vi "RTReedSwitch (1).vi"(8 "error in (no error)":errorcluster) -> (0 "error out":errorcluster)   [LabVIEW 2017]
uses:
  LoopPeriodGLOBAL.vi
  RTControl/StopGLOBAL.vi
  ReedSwitchDistanceGlobal.vi
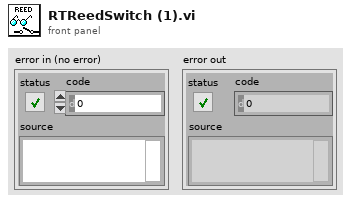
[diagram p1: front panel]
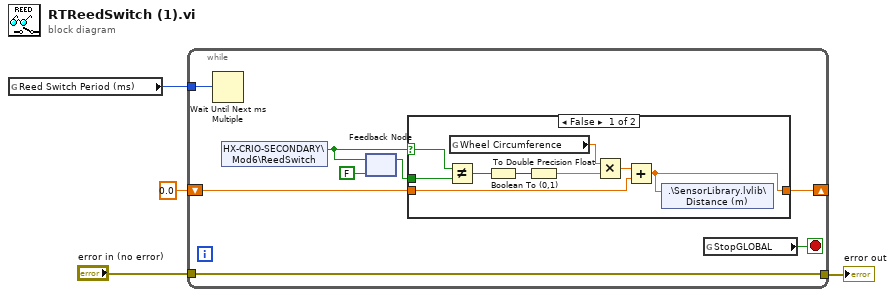
[diagram p0: block diagram]
diagram:
  n1 = global read "LoopPeriodGLOBAL.vi" "Reed Switch Period (ms)"() -> (w1:u32)
  n2 = while {
    shift-right: [w8] -> _
    shift-left: 0.0 -> [w12]
    tunnel: "error in (no error)" -> [w6]
    tunnel: [w6] -> w2
    tunnel: w1 -> [w5]
    stop <- w7 stop-if-true
    n3 = Wait Until Next ms Multiple(millisecond multiple=w5) -> ()  [unwired: 1 out]
    n4 = shared-variable "HX-CRIO-SECONDARY\\Mod6\\ReedSwitch"() -> (w11:bool)  [unwired: 1 in, 1 out]
    n5 = feedback-in #1(w11) -> ()
    n6 = feedback #1(FALSE) -> (w9:bool)
    n7 = case shown="False" w11 {
      selector: w11 -> [w21 _]
      tunnel: w12 -> [w16 w22]
      tunnel: w9 -> [w20 _]
      tunnel: [w13 w22] -> w8
      frame False {
        n8 = Not Equal?(x=w21, y=w20) -> (x != y?=w19:bool)
        n9 = global read "ReedSwitchDistanceGlobal.vi" "Wheel Circumference"() -> (w14:dbl)
        n10 = Boolean To (0,1)(Boolean=w19) -> (0, 1=w18:i16)
        n11 = To Double Precision Float(number=w18) -> (double precision float=w17:dbl)
        n12 = Multiply(x=w14, y=w17) -> (x*y=w15:dbl)
        n13 = Add(x=w15, y=w16) -> (x+y=w13:dbl)
        n14 = shared-variable ".\\SensorLibrary.lvlib\\Distance (m)"(w13) -> ()  [unwired: 1 in, 1 out]
      }
      frame True {
      }
    }
    n15 = global read "StopGLOBAL.vi" "StopGLOBAL"() -> (w7:bool)
  }
  "error out" <- w2
